vi "Log My Data CSV.vi"(6 "Data":waveform(dbl)={"t0"=timestamp(0 s since 1904-01-01), "dt"=0.0, "Y"=[]}, 8 "error in":errorcluster, 11 "file refnum":refnum<file>) -> (0 "error out":errorcluster, 3 "file refnum out":refnum<file>)   [LabVIEW 2014]
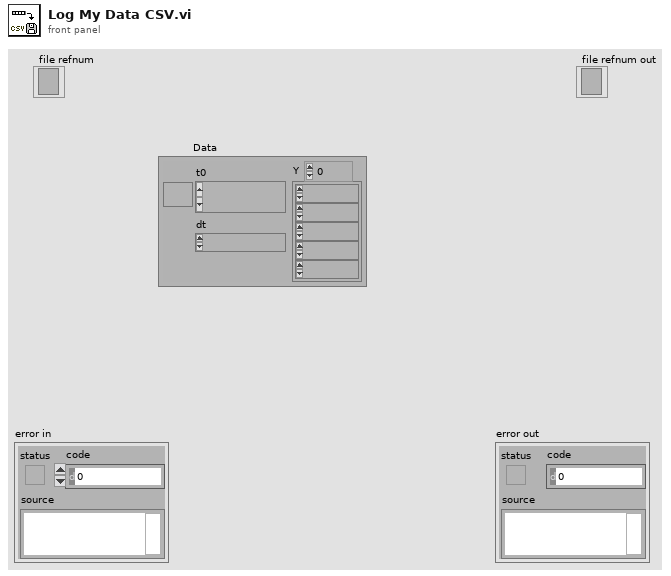
[diagram p1: front panel]
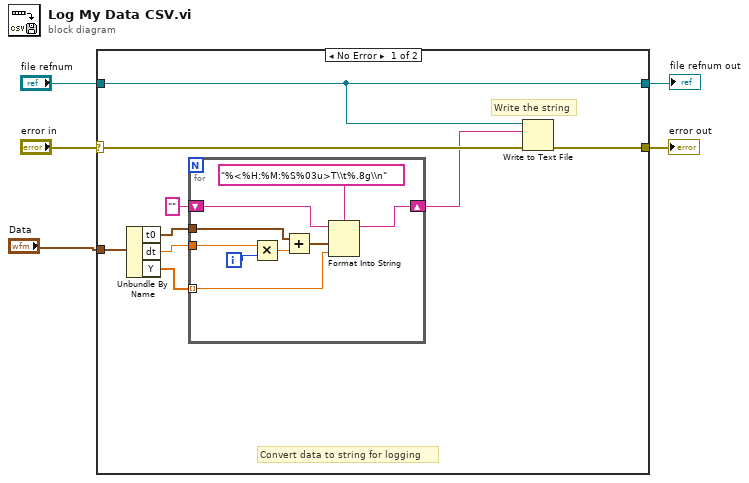
[diagram p0: block diagram]
diagram:
  n1 = case shown="No Error" "error in" {
    selector: "error in" -> [w13 w25]
    tunnel: "Data" -> [w11 _]
    tunnel: [w14 w25] -> w5
    tunnel: "file refnum" -> [w12 w24]
    tunnel: [w12 w24] -> w2
    frame No Error {
      # "Write the string"
      # "Convert data to string for logging"
      n2 = Unbundle By Name(w11) -> ("t0"=w8:timestamp, "dt"=w9:dbl, "Y"=w10:dbl[])
      n3 = for {
        tunnel: w10 -> [w15] mode=indexing
        tunnel: w9 -> [w23]
        tunnel: w8 -> [w20]
        shift-right: [w16] -> w6
        shift-left: "" -> [w17]
        i -> [w22]
        n4 = Multiply(x=w23, y=w22) -> (x*y=w21:dbl)
        n5 = Add(x=w20, y=w21) -> (x+y=w19:timestamp)
        n6 = Format Into String(format string="%<%H:%M:%S%03u>T\\t%.8g\\n", initial string=w17, w19, w15) -> (resulting string=w16:string)  [unwired: 1 in, 1 out]
      }
      n7 = Write to Text File(file (use dialog)=w12, text=w6, error in=w13) -> (error out=w14:errorcluster)  [unwired: 1 in, 2 out]
    }
    frame Error {
      # "Wire previous error through"
    }
  }
  "error out" <- w5
  "file refnum out" <- w2
